vi "Flush.vi"(8 "error in (no error)":errorcluster, 11 "YAML Parser in":refnum<class "YAML Parser.lvclass">) -> (0 "error out":errorcluster, 3 "YAML Parser out":refnum<class "YAML Parser.lvclass">)   [LabVIEW 2015, in "YAML Parser.lvclass"]
uses:
  YAML Parser.lvclass
  YAML Parser.lvclass/YAML Parser.ctl
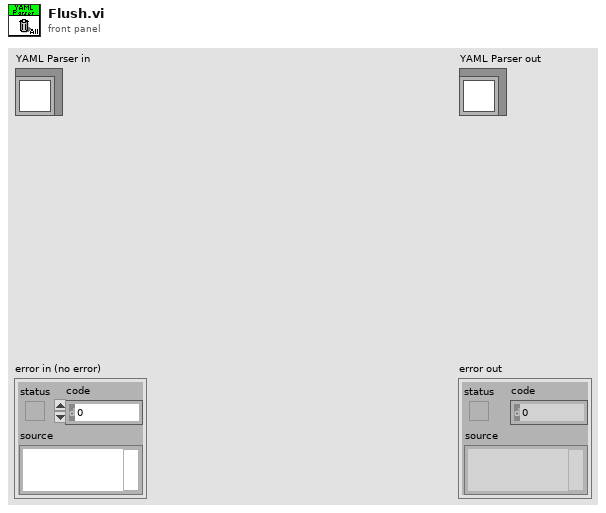
[diagram p1: front panel]
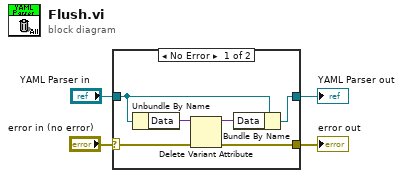
[diagram p0: block diagram]
diagram:
  n1 = case shown="No Error" "error in (no error)" {
    selector: "error in (no error)" -> [w7 w12]
    tunnel: [w6 w12] -> w3
    tunnel: [w10 w11] -> w1
    tunnel: "YAML Parser in" -> [w9 w11]
    frame No Error {
      n2 = Unbundle By Name(w9) -> ("Data"=w8:variant)
      n3 = Delete Variant Attribute(4:w7, 7:w8) -> (0:w6:errorcluster, 3:w5:variant)  [unwired: 1 in, 1 out]
      n4 = Bundle By Name(cluster=w9, "Data"=w5) -> (w10:refnum<class "YAML Parser.lvclass">)
    }
    frame Error {
    }
  }
  "error out" <- w3
  "YAML Parser out" <- w1
